vi "Get Class Data.vi"(7 "OwningVI":refnum<vi>, 11 "Class":variant) -> (2 "Can Access Members?":bool, 3 "Class Data":variant)   [LabVIEW 2020, in "TypeGraph.lvlib"]
uses:
  TypeGraph.lvlib
  <vilib>/Utility/Data Type/NI_Data Type.lvlib
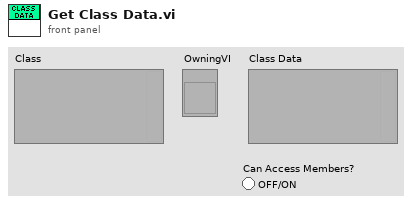
[diagram p1: front panel]
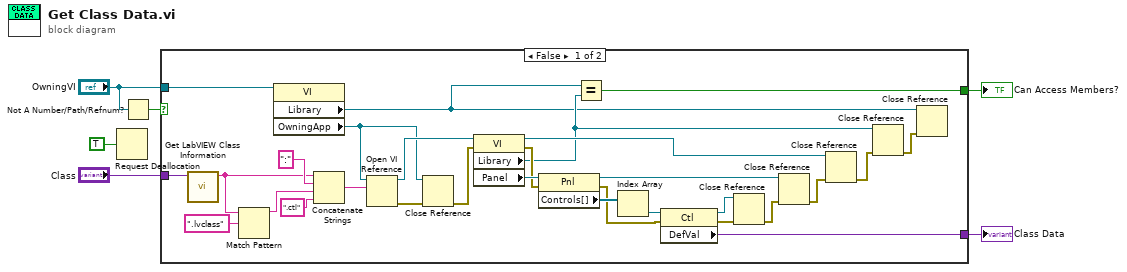
[diagram p0: block diagram]
diagram:
  n1 = Request Deallocation(TRUE ("flag")) -> ()
  n2 = Not A Number/Path/Refnum?(number/path/refnum="OwningVI") -> (NaN/Path/Refnum?=w1:bool)
  n3 = case shown="False" w1 {
    tunnel: "OwningVI" -> [w20 _]
    tunnel: "Class" -> [w19 _]
    tunnel: [w18 _] -> w5
    tunnel: [w11 _] -> w4
    frame False {
      n4 = call <vilib>:"Get LabVIEW Class Information.vi"("variant"=w19) -> ("LabVIEW class file name"=w21:string)  [unwired: 8 in, 2 out]
      n5 = Match Pattern(string=w21, regular expression=".lvclass") -> (before substring=w28:string)  [unwired: 1 in, 3 out]
      n6 = property class="VI"(reference=w20) -> ("Library"=w7:refnum<vi>, "OwningApp"=w23:refnum<vi>)  [unwired: 1 in, 2 out]
      n7 = Concatenate Strings(w21, ":" ("string"), w28, ".ctl" ("string")) -> (w22:string)
      n8 = Open VI Reference(application reference (local)=w23, vi path=w22) -> (vi reference=w26:refnum<vi>, error out=w25:errorcluster)  [unwired: 4 in]
      n9 = Close Reference(reference=w23, error in (no error)=w25) -> (error out=w24:errorcluster)
      n10 = property class="VI"(reference=w26, error in=w24) -> (reference out=w13:refnum<vi>, error out=w32:errorcluster, "Library"=w9:refnum<vi>, "Panel"=w35:refnum<vi>)
      n11 = property class="Pnl"(reference=w35, error in=w32) -> (reference out=w14:refnum<vi>, error out=w31:errorcluster, "Controls[]"=w34:refnum<vi>[])
      n12 = Equal?(x=w7, y=w9) -> (x = y?=w11:bool)
      n13 = Index Array(array=w34) -> (element=w33:refnum<vi>)  [unwired: 1 in]
      n14 = property class="Ctl"(reference=w33, error in=w31) -> (reference out=w16:refnum<vi>, error out=w17:errorcluster, "DefVal"=w18:variant)
      n15 = Close Reference(reference=w16, error in (no error)=w17) -> (error out=w15:errorcluster)
      n16 = Close Reference(reference=w14, error in (no error)=w15) -> (error out=w12:errorcluster)
      n17 = Close Reference(reference=w13, error in (no error)=w12) -> (error out=w10:errorcluster)
      n18 = Close Reference(reference=w9, error in (no error)=w10) -> (error out=w8:errorcluster)
      n19 = Close Reference(reference=w7, error in (no error)=w8) -> ()  [unwired: 1 out]
    }
    frame True {
    }
  }
  "Class Data" <- w5
  "Can Access Members?" <- w4
